vi "Begin.vi"(11 "Image Size":T1=enum."160x120") -> (0 "error out":errorcluster)   [LabVIEW 2012]
doc: "Called before other user functions, this VI is expected to open initial I/O refnums, load in file data, and do all program initialization. Notice that the <B>error out</B> terminal is simply used for data flow. Wiring it to other structures or subVIs ensures that this VI runs first."
uses:
  <vilib>/Rock Robotics/WPI/Camera/WPI_CameraImageSize.ctl
  <vilib>/Rock Robotics/WPI/Camera/WPI_CameraWhite Balance Values.ctl
  <vilib>/Rock Robotics/WPI/Camera/WPI_CameraExposure Values.ctl
  <vilib>/Rock Robotics/WPI/Camera/WPI_CameraFrameRate.ctl
  <vilib>/Rock Robotics/WPI/DriverStation/WPI_DriverStationRobotMode2.ctl
  <vilib>/Rock Robotics/WPI/Joystick/WPI_JoystickDeviceEnum.ctl
  <vilib>/Rock Robotics/SystemInterfaces/DIO/FPGA_DIOPWMChannel.ctl
  <vilib>/Rock Robotics/WPI/Solenoid/WPI_SolenoidChannel.ctl
  <vilib>/Rock Robotics/SystemInterfaces/Typedef/FPGA_TypedefSolenoidModule.ctl
  <vilib>/Rock Robotics/SystemInterfaces/Typedef/FPGA_TypedefAnalogModuleForGyro.ctl
  <vilib>/Rock Robotics/SystemInterfaces/AI/FPGA_AIGyroChannel.ctl
  <vilib>/Rock Robotics/SystemInterfaces/Typedef/FPGA_TypedefDigitalModule.ctl
  <vilib>/Rock Robotics/SystemInterfaces/DIO/FPGA_DIOChannel.ctl
  <vilib>/Rock Robotics/SystemInterfaces/DIO/FPGA_DIORelayChannel.ctl
  <vilib>/Rock Robotics/WPI/Encoder/WPI_EncoderType.ctl
  Robot Global Data.vi
  <vilib>/Rock Robotics/WPI/RobotDrive/WPI_RobotDriveOpen4MotorWithVictor.vi
  <vilib>/Rock Robotics/WPI/Solenoid/WPI_SolenoidOpenSingle.vi
  <vilib>/Rock Robotics/WPI/Solenoid/Deprecated/WPI_SolenoidSetBool.vi
  <vilib>/Rock Robotics/WPI/Compressor/WPI_CompressorGetSetRefNum.vi
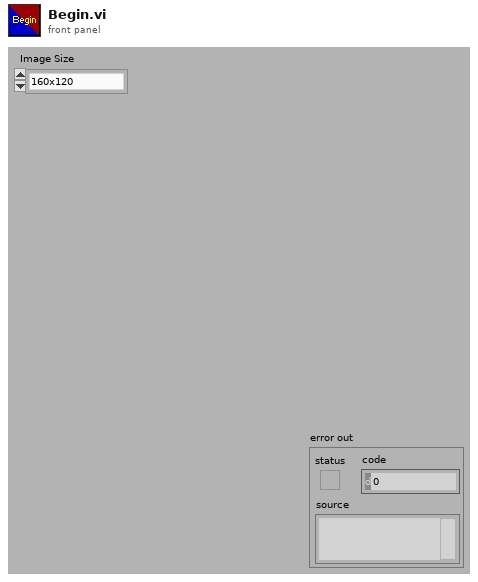
[diagram p1: front panel]
types:
  T1 = typedef "WPI_CameraImageSize.ctl" = enum16{"640x480", "320x240", "160x120"}
  T2 = typedef "WPI_EncoderType.ctl" = enum16{"1x", "2x", "4x"}
  T3 = typedef "FPGA_DIOChannel.ctl" = enum8{"DIO 1", "DIO 2", "DIO 3", "DIO 4", "DIO 5", "DIO 6", "DIO 7", "DIO 8", "DIO 9", "DIO 10", "DIO 11", "DIO 12", "DIO 13", "DIO 14", "Invalid"}
  T4 = typedef "FPGA_DIORelayChannel.ctl" = enum8{"Relay 1", "Relay 2", "Relay 3", "Relay 4", "Relay 5", "Relay 6", "Relay 7", "Relay 8", "Invalid"}
  T5 = typedef "FPGA_TypedefDigitalModule.ctl" = enum16{"Digital Module 1", "Digital Module 2"}
  T6 = typedef "FPGA_AIGyroChannel.ctl" = enum8{"AI 1", "AI 2", "Invalid"}
  T7 = typedef "FPGA_TypedefAnalogModuleForGyro.ctl" = enum16{"Analog Module 1"}
  T8 = typedef "FPGA_TypedefSolenoidModule.ctl" = enum16{"Solenoid Module 1", "Solenoid Module 2"}
  T9 = typedef "WPI_SolenoidChannel.ctl" = enum8{"Solenoid 1", "Solenoid 2", "Solenoid 3", "Solenoid 4", "Solenoid 5", "Solenoid 6", "Solenoid 7", "Solenoid 8", "Invalid"}
  T10 = typedef "FPGA_DIOPWMChannel.ctl" = enum8{"PWM 1", "PWM 2", "PWM 3", "PWM 4", "PWM 5", "PWM 6", "PWM 7", "PWM 8", "PWM 9", "PWM 10", "Invalid"}
  T11 = typedef "WPI_JoystickDeviceEnum.ctl" = enum16{"USB 1", "USB 2", "USB 3", "USB 4", "Kinect 1", "Kinect 2"}
  T12 = typedef "WPI_DriverStationRobotMode2.ctl" = enum16{"Autonomous Disabled", "Autonomous Enabled", "Teleop Disabled", "Teleop Enabled", "Timeout", "Finish", "Test Disabled", "Test Enabled"}
  T13 = typedef "WPI_CameraFrameRate.ctl" = u32
  T14 = typedef "WPI_CameraExposure Values.ctl" = enum16{"Auto", "Flicker-free 50 Hz", "Flicker-free 60 Hz", "Hold current"}
  T15 = typedef "WPI_CameraWhite Balance Values.ctl" = enum16{"Auto", "Fixed indoor", "Fixed outdoor 1", "Fixed outdoor 2", "Fixed fluorescent 1", "Fixed fluorescent 2", "Hold current"}
  T16 = typedef "WPI_CompressorDevRef.ctl" = cluster{"DevStatus":errorcluster, "DigitalInputDevRef":T17, "RelayDevRef":T18}
  T17 = typedef "WPI_DigitalInputDevRef.ctl" = cluster{"DevStatus":errorcluster, "DIO Channel":T3, "Digital Module":T5}
  T18 = typedef "WPI_RelayDevRef.ctl" = cluster{"DevStatus":errorcluster, "Relay Channel":T4, "Digital Module":T5, "Relay Direction":T19}
  T19 = typedef "WPI_RelayDirection.ctl" = enum16{"Both directions", "Forward only", "Reverse only"}
  T20 = typedef "FPGA_CounterEncoderSourceConvertionLVSourceType.ctl" = cluster{"DevStatus":errorcluster, "AnalogTriggerMode?":bool, "DigitalMode":cluster{"Digital Module":T5, "DIO Channel":T21}, "AnalogTriggerMode":cluster{"AnalogTriggerIndex":T22, "OutputType":T23}}
  T21 = typedef "FPGA_DIODigitalSourceChannel.ctl" = enum8{"DIO 1", "DIO 2", "DIO 3", "DIO 4", "DIO 5", "DIO 6", "DIO 7", "DIO 8", "DIO 9", "DIO 10", "DIO 11", "DIO 12", "DIO 13", "DIO 14", "Disabled"}
  T22 = typedef "FPGA_AnalogTriggerIndex.ctl" = enum8{"Trig 0", "Trig 1", "Trig 2", "Trig 3", "Trig 4", "Trig 5", "Trig 6", "Trig 7", "Invalid"}
  T23 = typedef "FPGA_AnalogTriggerOutType.ctl" = enum16{"InWindow", "TriggerState", "Rising", "Falling"}
  T24 = typedef "WPI_JoystickDevRef.ctl" = cluster{"Device":T11}
  T25 = typedef "WPI_GyroDevRef.ctl" = cluster{"DevStatus":errorcluster, "Analog Module":T26, "Analog Channel":T27, "Offset":dbl, "Gain (VoltsPerDegree/Second)":dbl}
  T26 = typedef "FPGA_TypedefAnalogModule.ctl" = enum16{"Analog Module 1", "Analog Module 2"}
  T27 = typedef "FPGA_AIChannel.ctl" = enum8{"AI 1", "AI 2", "AI 3", "AI 4", "AI 5", "AI 6", "AI 7", "AI 8", "Invalid"}
  T28 = typedef "WPI_SolenoidDevRef.ctl" = cluster{"DevStatus":errorcluster, "Solenoid Module":T8, "Forward Solenoid Channel":T9, "Reverse Solenoid Channel":T9}
  T29 = typedef "WPI_CameraDevRef.ctl" = cluster{"Camera Address":string, "CameraStatus":errorcluster, "Acquire Image Notifier":refnum<notifier>}
  T30 = typedef "WPI_EncoderDevRef.ctl" = cluster{"DevStatus":errorcluster, "EncoderIndex":T31, "CounterIndex":T32, "DistancePerCount":dbl, "Decoding Type":T2}
  T31 = typedef "FPGA_EncoderIdx.ctl" = enum8{"Enc 0", "Enc 1", "Enc 2", "Enc 3", "Invalid"}
  T32 = typedef "FPGA_CounterCtrSystemIndex.ctl" = enum8{"Ctr 0", "Ctr 1", "Ctr 2", "Ctr 3", "Ctr 4", "Ctr 5", "Ctr 6", "Ctr 7", "Invalid"}
  T33 = typedef "WPI_RobotDriveDevRef.ctl" = cluster{"DevStatus":errorcluster, "Motors[]":T34[], "Square Inputs":bool, "Max Output":dbl, "Isochronous":bool}
  T34 = typedef "WPI_MotorControlDeviceRef.ctl" = cluster{"DeviceStatus":errorcluster, "Type":enum16{"PWM", "CAN"}, "PWM":cluster{"Digital Module":T5, "PWM Channel":T10, "DeadBand":T35}, "CAN":cluster{"Device Number":u8, "Control Mode":T36, "Semaphore":T37, "Max Vout":dbl}, "Invert":bool, "TransformRef":T38, "InvTransformRef":T38}
  T35 = typedef "WPI_PWMDeadband.ctl" = cluster{"Name":string, "maxPositivePwm":i32, "minPositivePwm":i32, "centerPwm":i32, "maxNegativePwm":i32, "minNegativePwm":i32, "angularRange":u16}
  T36 = typedef "WPI_CANJaguar_ControlMode.ctl" = enum8{"Percent VBus", "Current", "Speed", "Position", "Voltage"}
  T37 = typedef "Semaphore RefNum" = refnum<k1>
  T38 = typedef "WPI_PWMTransform_ConPane.ctl" = refnum<vi>
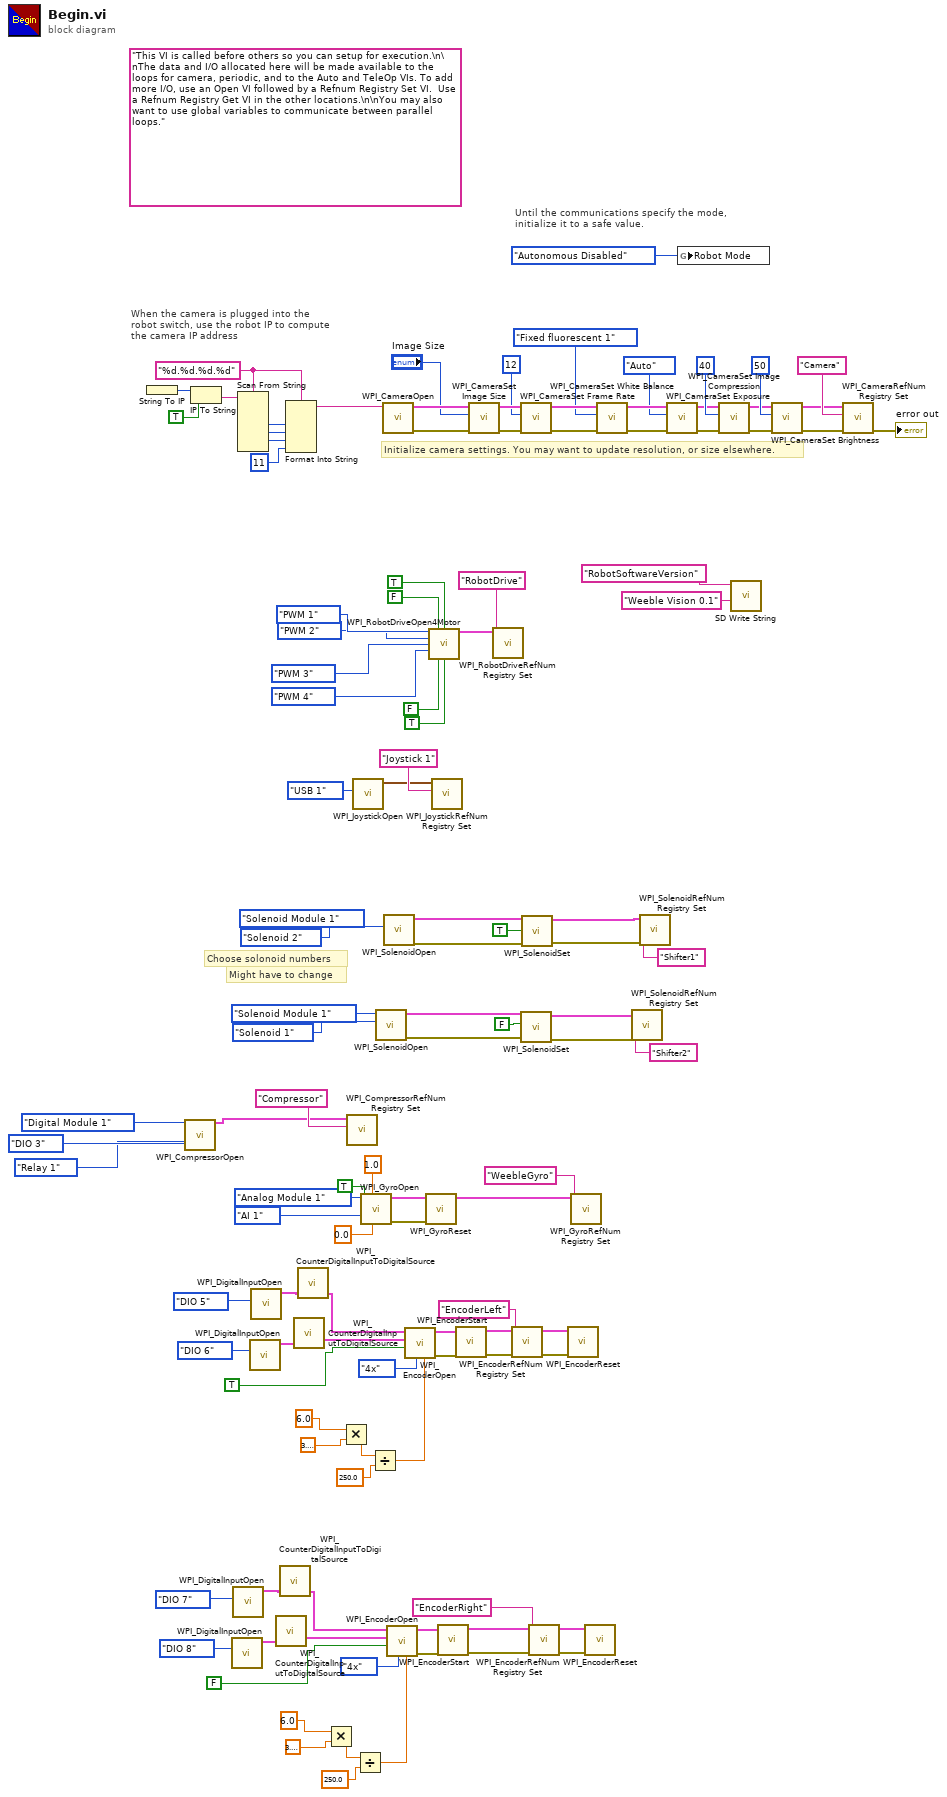
[diagram p0: block diagram]
diagram:
  (unwired) FPGA_TypedefSolenoidModule."Solenoid Module 1" ("Solenoid Module (Module 1)")
  w88 = "%d.%d.%d.%d" ("format string")
  (unwired) "This VI is called before others so you can setup for execution.\n\nThe data and I/O allocated here will be made available to the loops for camera, periodic, and to the Auto and TeleOp VIs. To add more I/O, use an Open VI followed by a Refnum Registry Set VI.  Use a Refnum Registry Get VI in the other locations.\n\nYou may also want to use global variables to communicate between parallel loops."
  # "Might have to change"
  # "Choose solonoid numbers"
  # "Until the communications specify the mode,\ninitialize it to a safe value."
  # "When the camera is plugged into the\nrobot switch, use the robot IP to compute\nthe camera IP address"
  # "Initialize camera settings. You may want to update resolution, or size elsewhere."
  n1 = String To IP() -> (0:w95:u32)  [unwired: 1 in]
  n2 = call <vilib>:"WPI_CompressorOpen.vi"("Pressure Switch Digital Module (Module 1)"=FPGA_TypedefDigitalModule."Digital Module 1" ("Pressure Switch DIO Module"), "Pressure Switch DIO Channel"=FPGA_DIOChannel."DIO 3", "Relay Channel"=FPGA_DIORelayChannel."Relay 1") -> ("CompressorDevRef"=w50:T16)  [unwired: 2 in, 10 out]
  n3 = IP To String(1:TRUE ("dot notation? (F)"), 2:w95) -> (0:w93:string)
  n4 = call <vilib>:"WPI_DigitalInputOpen.vi"("DIO Channel"=FPGA_DIOChannel."DIO 8" ("B Channel")) -> ("DigitalInputDevRef"=w18:T17)  [unwired: 2 in, 8 out]
  n5 = call <vilib>:"WPI_DigitalInputOpen.vi"("DIO Channel"=FPGA_DIOChannel."DIO 7" ("A Channel")) -> ("DigitalInputDevRef"=w20:T17)  [unwired: 2 in, 8 out]
  n6 = Scan From String(format string=w88, input string=w93) -> (output 1=w92:i32, output 2=w91:i32, output 3=w90:i32)  [unwired: 7 in, 3 out]
  n7 = call <vilib>:"WPI_DigitalInputOpen.vi"("DIO Channel"=FPGA_DIOChannel."DIO 6" ("B Channel")) -> ("DigitalInputDevRef"=w33:T17)  [unwired: 2 in, 8 out]
  n8 = call <vilib>:"WPI_DigitalInputOpen.vi"("DIO Channel"=FPGA_DIOChannel."DIO 5" ("A Channel")) -> ("DigitalInputDevRef"=w35:T17)  [unwired: 2 in, 8 out]
  n9 = call <vilib>:"WPI_CounterDigitalInputToDigitalSource.vi"("DigitalInputDevRef"=w18) -> ("Digital Source"=w24:T20)  [unwired: 6 out]
  n10 = call <vilib>:"WPI_CounterDigitalInputToDigitalSource.vi"("DigitalInputDevRef"=w20) -> ("Digital Source"=w22:T20)  [unwired: 6 out]
  n11 = Format Into String(format string=w88, w92, w91, w90, 11 ("Compression")) -> (resulting string=w86:string)  [unwired: 2 in, 1 out]
  n12 = call <vilib>:"WPI_CounterDigitalInputToDigitalSource.vi"("DigitalInputDevRef"=w33) -> ("Digital Source"=w39:T20)  [unwired: 6 out]
  n13 = call <vilib>:"WPI_CounterDigitalInputToDigitalSource.vi"("DigitalInputDevRef"=w35) -> ("Digital Source"=w37:T20)  [unwired: 6 out]
  n14 = Multiply(x=6.0 ("DistancePerCount"), y=3.141592653589793) -> (x*y=w6:dbl)
  n15 = Multiply(x=6.0 ("DistancePerCount"), y=3.141592653589793) -> (x*y=w10:dbl)
  n16 = call <vilib>:"WPI_CompressorRefNum Registry Set.vi"("refnum name"="Compressor", "CompressorDevRef"=w50) -> ()  [unwired: 1 in, 9 out]
  n17 = call <vilib>:"WPI_JoystickOpen.vi"("JoystickDevice"=WPI_JoystickDeviceEnum."USB 1") -> ("JoystickDevRef"=w84:T24)  [unwired: 10 in]
  n18 = Divide(x=w6, y=250.0 ("DistancePerCount")) -> (x/y=w3:dbl)
  n19 = call <vilib>:"WPI_GyroOpen.vi"("Calibrated Center Voltage"=0.0, "Calibration Time (s)"=1.0, "Calibrate On Open"=TRUE, "Analog Channel"=FPGA_AIGyroChannel."AI 1", "Analog Module (Module 1)"=FPGA_TypedefAnalogModuleForGyro."Analog Module 1") -> ("error out"=w52:errorcluster, "GyroDevRef"=w56:T25)  [unwired: 4 in, 1 out]
  n20 = Divide(x=w10, y=250.0 ("DistancePerCount")) -> (x/y=w8:dbl)
  n21 = call-poly <vilib>:"WPI_SolenoidOpen.vi"("Solenoid Channel"=WPI_SolenoidChannel."Solenoid 1", "Solenoid Module (Module 1)"=FPGA_TypedefSolenoidModule."Solenoid Module 1") -> ("error out"=w60:errorcluster, "SolenoidDevRef"=w62:T28)  [unwired: 8 in]
  n22 = call <vilib>:"WPI_CameraOpen.vi"("Camera Address"=w86) -> ("error out"=w107:errorcluster, "CameraDevRef"=w108:T29)  [unwired: 1 in, 8 out]
  n23 = call-poly <vilib>:"WPI_SolenoidOpen.vi"("Solenoid Channel"=WPI_SolenoidChannel."Solenoid 2") -> ("error out"=w65:errorcluster, "SolenoidDevRef"=w58:T28)  [unwired: 9 in]
  n24 = call <vilib>:"WPI_EncoderOpen.vi"("DistancePerCount"=w3, "Decoding Type"=WPI_EncoderType."4x", "Invert Direction (False)"=FALSE ("Invert Direction"), "BSource"=w24, "ASource"=w22) -> ("error out"=w15:errorcluster, "EncoderDevRef"=w25:T30)  [unwired: 3 in, 2 out]
  n25 = call <vilib>:"WPI_EncoderOpen.vi"("DistancePerCount"=w8, "Decoding Type"=WPI_EncoderType."4x", "Invert Direction (False)"=TRUE ("Invert Direction"), "BSource"=w39, "ASource"=w37) -> ("error out"=w30:errorcluster, "EncoderDevRef"=w40:T30)  [unwired: 3 in, 2 out]
  n26 = call <vilib>:"WPI_GyroReset.vi"("error in (no error)"=w52, "GyroDevRef"=w56) -> ("GyroDevRef"=w46:T25)  [unwired: 8 in, 1 out]
  n27 = call-poly <vilib>:"WPI_RobotDriveOpen4Motor.vi"("Rear Left Motor"=FPGA_DIOPWMChannel."PWM 1", "Rear Left Motor Inverted"=FALSE, "Rear Right Motor Inverted"=TRUE, "Rear Right Motor"=FPGA_DIOPWMChannel."PWM 2", "Front Left Motor"=FPGA_DIOPWMChannel."PWM 3", "Front Right Motor"=FPGA_DIOPWMChannel."PWM 4" ("Front Left Motor"), "Front Left Motor Inverted"=FALSE, "Front Right Motor Inverted"=TRUE) -> ("RobotDriveDevRef"=w73:T33)  [unwired: 6 in, 1 out]
  n28 = call <vilib>:"WPI_JoystickRefNum Registry Set.vi"("refnum name"="Joystick 1", "JoystickDevRef"=w84) -> ()  [unwired: 8 in, 2 out]
  n29 = call <vilib>:"WPI_EncoderStart.vi"("error in (no error)"=w15, "EncoderDevRef"=w25) -> ("error out"=w17:errorcluster, "EncoderDevRef"=w16:T30)  [unwired: 8 out]
  n30 = call <vilib>:"WPI_EncoderStart.vi"("error in (no error)"=w30, "EncoderDevRef"=w40) -> ("error out"=w32:errorcluster, "EncoderDevRef"=w31:T30)  [unwired: 8 out]
  n31 = call <vilib>:"WPI_CameraSet Image Size.vi"("error in (no error)"=w107, "Image Size"="Image Size", "CameraDevRef"=w108) -> ("error out"=w106:errorcluster, "CameraDevRef Out"=w109:T29)  [unwired: 7 out]
  n32 = call <vilib>:"WPI_RobotDriveRefNum Registry Set.vi"("refnum name"="RobotDrive", "RobotDriveDevRef"=w73) -> ()  [unwired: 8 in, 2 out]
  n33 = call <vilib>:"WPI_EncoderRefNum Registry Set.vi"("error in (no error)"=w32, "refnum name"="EncoderLeft", "EncoderDevRef"=w31) -> ("error out"=w42:errorcluster, "EncoderDevRef"=w41:T30)  [unwired: 7 out]
  n34 = call <vilib>:"WPI_CameraSet Frame Rate.vi"("error in (no error)"=w106, "Frame Rate (fps)"=T13 12, "CameraDevRef"=w109) -> ("error out"=w105:errorcluster, "CameraDevRef Out"=w111:T29)  [unwired: 7 out]
  n35 = call-poly <vilib>:"WPI_SolenoidSet.vi"("error in (no error)"=w60, "Value"=FALSE, "SolenoidDevRef"=w62) -> ("error out"=w59:errorcluster, "SolenoidDevRef"=w61:T28)  [unwired: 7 in]
  n36 = call-poly <vilib>:"WPI_SolenoidSet.vi"("error in (no error)"=w65, "Value"=TRUE, "SolenoidDevRef"=w58) -> ("error out"=w66:errorcluster, "SolenoidDevRef"=w57:T28)  [unwired: 7 in]
  n37 = call <vilib>:"WPI_EncoderRefNum Registry Set.vi"("error in (no error)"=w17, "refnum name"="EncoderRight", "EncoderDevRef"=w16) -> ("error out"=w27:errorcluster, "EncoderDevRef"=w26:T30)  [unwired: 7 out]
  n38 = call <vilib>:"WPI_EncoderReset.vi"("error in (no error)"=w42, "EncoderDevRef"=w41) -> ()  [unwired: 10 out]
  n39 = call <vilib>:"WPI_GyroRefNum Registry Set.vi"("refnum name"="WeebleGyro", "GyroDevRef"=w46) -> ()  [unwired: 8 in, 2 out]
  n40 = call <vilib>:"WPI_EncoderReset.vi"("error in (no error)"=w27, "EncoderDevRef"=w26) -> ()  [unwired: 10 out]
  n41 = call <vilib>:"WPI_CameraSet White Balance.vi"("error in (no error)"=w105, "White Balance"=WPI_CameraWhite_Balance_Values."Fixed fluorescent 1", "CameraDevRef"=w111) -> ("error out"=w104:errorcluster, "CameraDevRef Out"=w110:T29)  [unwired: 7 out]
  n42 = call <vilib>:"WPI_SolenoidRefNum Registry Set.vi"("error in (no error)"=w59, "refnum name"="Shifter2", "SolenoidDevRef"=w61) -> ()  [unwired: 7 in, 2 out]
  n43 = call <vilib>:"WPI_SolenoidRefNum Registry Set.vi"("error in (no error)"=w66, "refnum name"="Shifter1", "SolenoidDevRef"=w57) -> ()  [unwired: 7 in, 2 out]
  n44 = call <vilib>:"WPI_CameraSet Exposure.vi"("error in (no error)"=w104, "Exposure"=WPI_CameraExposure_Values."Auto", "CameraDevRef"=w110) -> ("error out"=w103:errorcluster, "CameraDevRef Out"=w113:T29)  [unwired: 7 out]
  n45 = global write "Robot Global Data.vi" "Robot Mode"(WPI_DriverStationRobotMode2."Autonomous Disabled" ("Robot Mode")) -> ()
  n46 = call <vilib>:"WPI_CameraSet Image Compression.vi"("error in (no error)"=w103, "Compression"=40, "CameraDevRef"=w113) -> ("error out"=w102:errorcluster, "CameraDevRef Out"=w112:T29)  [unwired: 7 out]
  n47 = call <vilib>:"SD Write String.vi"("String"="Weeble Vision 0.1", "Name"="RobotSoftwareVersion") -> ()  [unwired: 8 in, 2 out]
  n48 = call <vilib>:"WPI_CameraSet Brightness.vi"("error in (no error)"=w102, "Brightness"=50, "CameraDevRef"=w112) -> ("error out"=w100:errorcluster, "CameraDevRef Out"=w101:T29)  [unwired: 7 out]
  n49 = call <vilib>:"WPI_CameraRefNum Registry Set.vi"("error in (no error)"=w100, "refnum name"="Camera", "CameraDevRef"=w101) -> ("error out"=→"error out":errorcluster)  [unwired: 8 out]
